vi "Main_2018-02-09.vi"() -> ()   [LabVIEW 2017, in "Client.lvlib"]
uses:
  Client.lvlib
  ClientErrorHandler/ErrorLoopInitData.ctl
  ServerCommunications/TypeDefs/ClientConfiguration.ctl
  ParserSorter/SR Data.ctl
  ParserSorter/AE Group.ctl
  ParserSorter/SR Status.ctl
  ParserSorter/SR Level.ctl
  ParserSorter/SR Type.ctl
  CommunicationsFrameWork/TypeDefs/InternalData.ctl
  ServerCommunications/TypeDefs/SR List.ctl
  ServerCommunications/TypeDefs/SR Data.ctl
  ServerCommunications/TypeDefs/Connection Status.ctl
  UI_API/UIReferences.ctl
  UI_API/SR Fields.ctl
  CommunicationsFrameWork/CommsFrameWork.lvlib
  ServerCommunications/CommsServer.lvlib
  <vilib>/httpClient/LabVIEWHTTPClient.lvlib
  ClientErrorHandler/ClientErrorHandler.lvlib
  ClientLogger/ClientLogger.lvlib
  ParserSorter/ParserSorter.lvlib
  UI_API/UI_API.lvlib
panel:
  out "Prio 4":u32(colorbox)
  out "Prio 3":u32(colorbox)
  out "Prio 2":u32(colorbox)
  out "Prio 1":u32(colorbox)
  in  "Filter Preset":T1(ring)
  out "Time to Refresh":dbl(slide) scale=0.0..10.0
  out "Connection Quality":dbl(knob) scale=0.0..10.0
  out "Connected?":bool
  out "Last Update":timestamp
  in  "Refresh":bool
  in  "AE Level":enum16{"AE / ELP", "AE Intern"}(ring)
  in  "AE Groups":i32[](listbox)
  in  "SRs Tab":enum32{"Unassigned", "Assigned", "Debug"}(tab)
  out "Unassigned Sorted SRs":string[][](table)
  out "Assigned Sorted SRs":string[][](table)
  out "Last Error":errorcluster
  in  "Text":string="Manual Log Entry"
  in  "Type":string="Event"
  in  "Generate Log Entry":bool
  in  "Injected Error":errorcluster
  in  "Generate Error":bool
  # "Priority 1"
  # "Priority 3"
  # "Priority 2"
  # "Priority 4"
  # "Heartbeat Communication"
  # "Manual Loop Control"
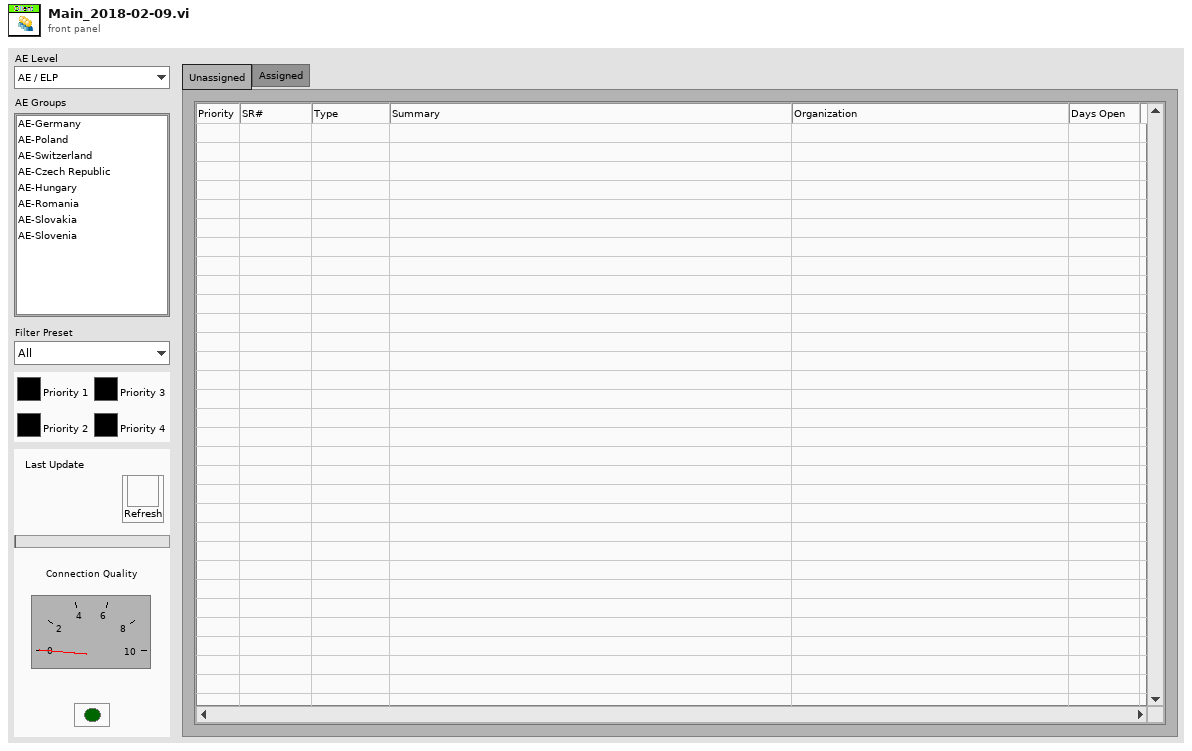
[diagram p1: front panel]
types:
  T1 = enum16{"All", "Eastern Europe", "DACH", "Custom"}
  T2 = typedef "Client.lvlib/CommsFrameWork.lvlib/CommReferences.ctl" = cluster{"ErrorEventReg":refnum<event-registration>, "ErrorEvent":refnum<user-event>, "Queues":cluster{"MHLClient":refnum<queue>, "ErrorHandler":refnum<queue>, "EventHandler":refnum<queue>, "ConnectionHandler":refnum<queue>, "UIHandler":refnum<queue>, "Logger":refnum<queue>}}
  T3 = typedef "LVPoint32TypeDef.ctl" = cluster{"Horizontal":i32, "Vertical":i32}
  T4 = typedef "Client.lvlib/UI_API.lvlib/UIReferences.ctl" = cluster{"Assigned SRs":refnum<vi>, "Unassigned SRs":refnum<vi>, "AE Level":refnum<vi>, "AE Groups":refnum<vi>}
  T5 = typedef "Client.lvlib/ParserSorter.lvlib/SR Data.ctl" = cluster{"SR Number":i64, "AE Group":T6, "SR Owner":string, "Summary":string, "SR Status":T7, "Days Open":dbl, "Prio":T8, "SR Type":T9, "Service Level":string, "Last Updated":timestamp, "First Name":string, "Last Name":string, "Organisation Name":string, "Creation Date":timestamp, "Needs Merging?":bool, "English Flag?":bool}
  T6 = typedef "Client.lvlib/ParserSorter.lvlib/AE Group.ctl" = enum32{"NaN", "AE-Germany", "AE-Poland", "AE-Switzerland", "AE-Czech Republic", "AE-Hungary", "AE-Romania", "AE-Slovakia", "AE-Slovenia"}
  T7 = typedef "Client.lvlib/ParserSorter.lvlib/SR Status.ctl" = enum32{"NaN", "Caller Abandoned", "Created in Error", "Declined to Purchase Support", "Expired", "Forum Resolved AE", "Forum Resolved Customer", "IN WORK", "IN WORK Collab with AES", "IN WORK Collab with PSE", "IN WORK Collab with SE", "IN WORK Escalation", "IN WORK Customer Added Note", "Open", "Potentially Resolved", "POC Resolved", "Resolved", "RMA Waiting on Customer", "RMA Open", "RMA In Progress", "RMA Closed - DOA", "RMA Closed", "RMA Approved for Return", "Project Complete", "Presumed Resolved", "IN WORK Wait on Customer"}
  T8 = typedef "Client.lvlib/ParserSorter.lvlib/SR Level.ctl" = enum16{"Prio 1", "Prio 2", "Prio 3", "Prio 4"}
  T9 = typedef "Client.lvlib/ParserSorter.lvlib/SR Type.ctl" = enum32{"NaN", "ATE Core Configurations (BYOATE)", "Activation", "BioBench", "CAN", "CM C Series", "Calibration", "Consulting Services", "CounterTimer", "DAQExpress", "DASYLab", "DIAdem", "DMM", "DSA HW", "Digital_IO", "FIRST (NIC Only)", "FieldBus", "FieldPoint", "Functional Savety", "GATI", "GPIB", "HMI and Industrial PCs", "HiQ", "HighSpeedDigital_IO", "IMAQ", "IOTech Vibration", "Industrial Communications", "InsightCM", "LV", "LV CD&Sim", "LV Comms", "LV Controls Add-Ons", "LV Embedded", "LV MathScript RT", "LV NXG", "LV NXT", "LVDSC", "LVFPGA", "LVPDA and LV Touch Panel", "LVRT", "LabWindows_CVI", "Lookout", "MATRIXx", "MStudioDotNet", "MStudioVisualBasic", "MStudioVisualC", "Measure (Legacy)", "Motion", "MultifunctionDAQ", "Multimedia Test HW/SW", "Multisim (EWB)", "NI Update Service", "OPC Servers", "Optical (OSI)", "PXI Controllers, Chassis, MXI", "PXI Timing and Sync", "Power Supplies and SMUs", "Powertrain Controls", "RAID", "RF", "RF Software", "RIO", "SC Express", "SCC", "SCXI", "SPEEDY-33 (Hyperception)", "STS", "ScopeDigitizers", "Serial", "Signal Sources", "SignalCondOther", "SignalExpress", "Software Defined Intruments", "Sound and Vibration SW", "Switch Executive", "Switches", "TestStand", "USRP", "Ultiboard (EWB)", "VBench", "VI Logger", "VXI_MXI", "VeriStand", "VisionSW", "VolumeLicenseMgr", "WSN", "Web UI Builder", "myRIO"}
  T10 = typedef "Client.lvlib/CommsServer.lvlib/Connection Status.ctl" = cluster{"Connection Quality":dbl, "Last Update":timestamp}
  T11 = typedef "Client.lvlib/ParserSorter.lvlib/SR Fields.ctl" = enum16{"SR Number", "AE Group", "SR Owner", "Summary", "SR Status", "Days Open", "Prio", "SR Type", "Service Level", "Last Updated", "First Name", "Last Name", "Organisation Name", "Creation Date", "Needs Merging?", "English Flag?"}
  T12 = typedef "Client.lvlib/CommsServer.lvlib/ClientConfiguration.ctl" = cluster{"ColorCodes":u32[]}
  T13 = typedef "Client.lvlib/ClientErrorHandler.lvlib/ErrorLoopInitData.ctl" = cluster{"ErrorsToIgnore":i32[]}
  T14 = typedef "Client.lvlib/CommsFrameWork.lvlib/InternalData.ctl" = cluster{"Connection Data":cluster{"IP":string, "Port":string, "ClientName":string}}
  T15 = typedef "Client.lvlib/CommsServer.lvlib/SR List.ctl" = T16[]
  T16 = typedef "Client.lvlib/CommsServer.lvlib/SR Data.ctl" = cluster{"SR#":dbl, "Group":string, "Owner":string, "Problem Summary":string, "Last Updated":timestamp, "Customer First Name":string, "Customer Last Name":string, "Company":string, "Created On":timestamp, "SR Type":string, "Status":string, "Service Level":string, "Channel":string, "Days Open":dbl}
  T17 = cluster{"IP":string, "Port":string, "ClientName":string}
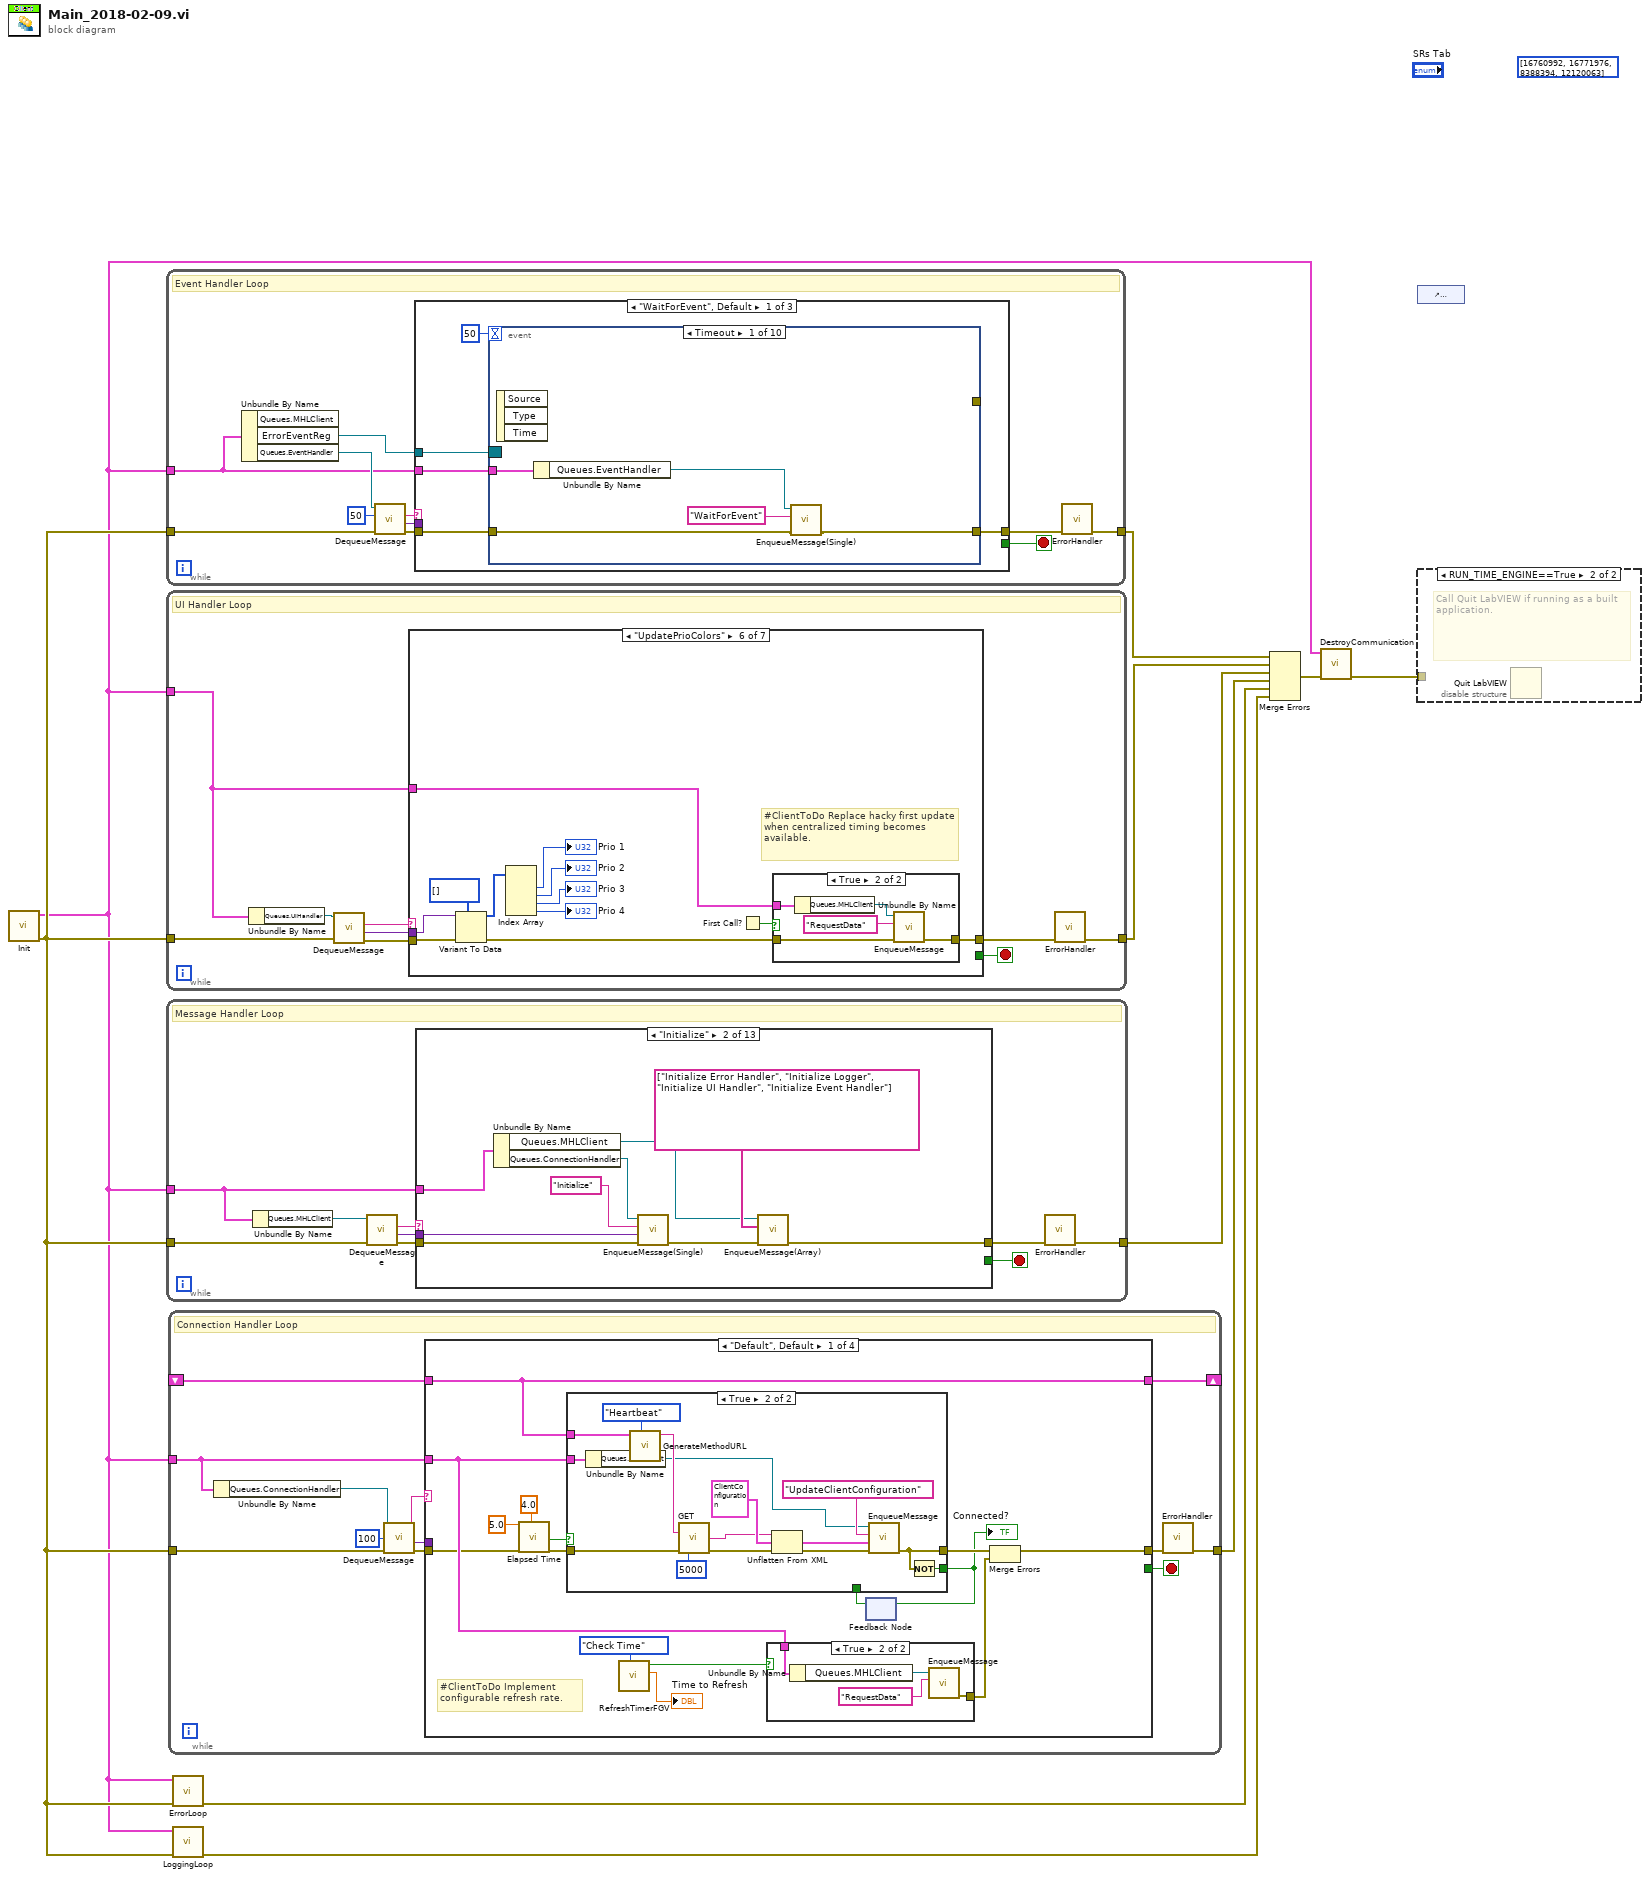
[diagram p0: block diagram]
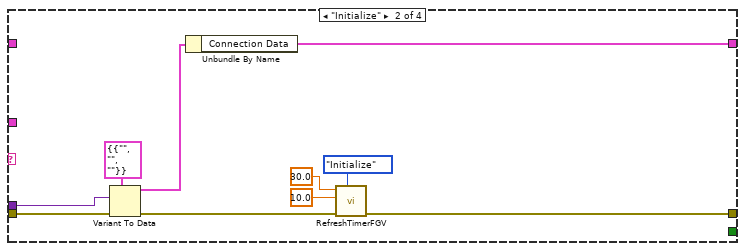
[diagram p4: hidden frame]
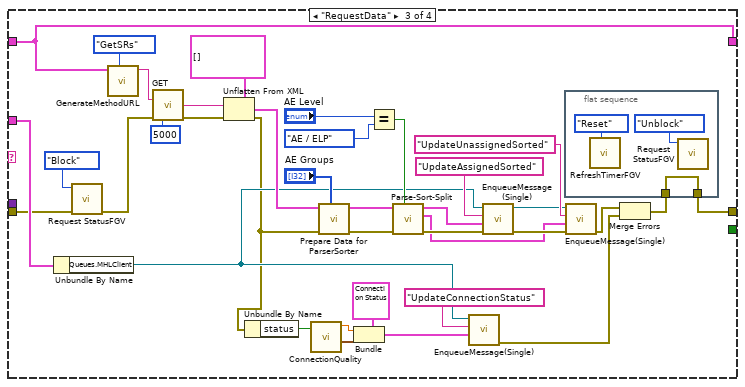
[diagram p5: hidden frame]
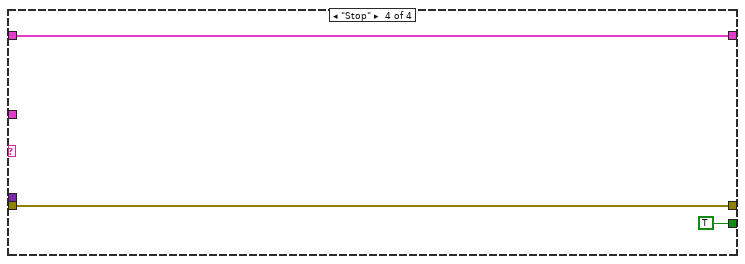
[diagram p6: hidden frame]
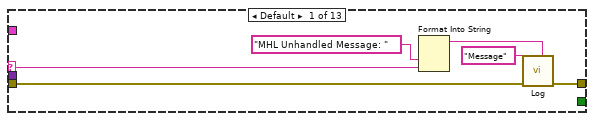
[diagram p7: hidden frame]
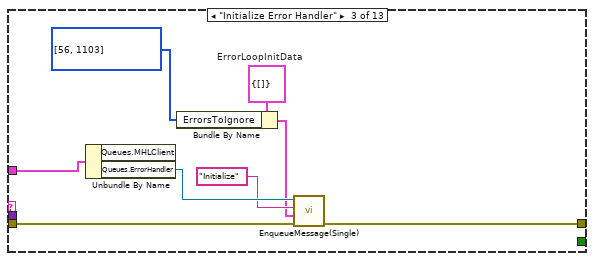
[diagram p8: hidden frame]
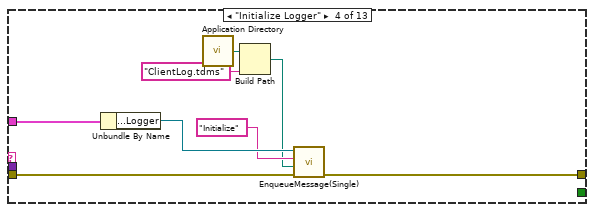
[diagram p9: hidden frame]
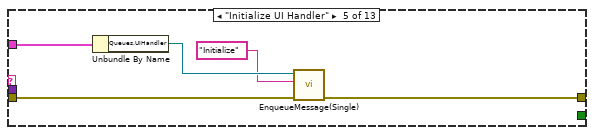
[diagram p10: hidden frame]
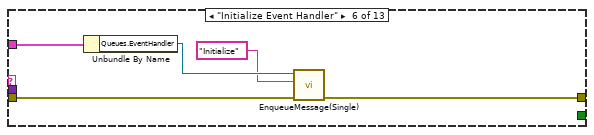
[diagram p11: hidden frame]
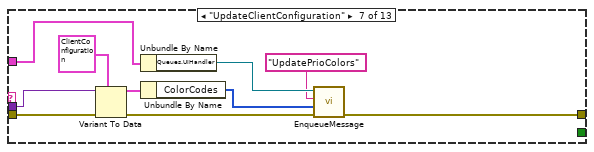
[diagram p12: hidden frame]
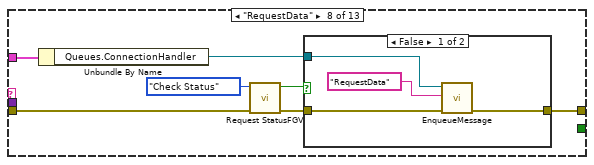
[diagram p13: hidden frame]
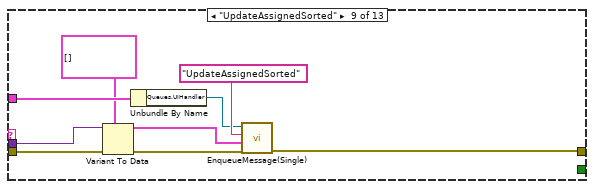
[diagram p15: hidden frame]
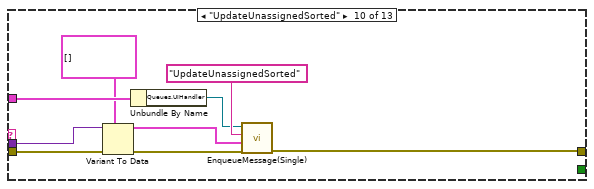
[diagram p16: hidden frame]
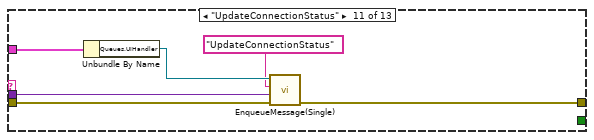
[diagram p17: hidden frame]
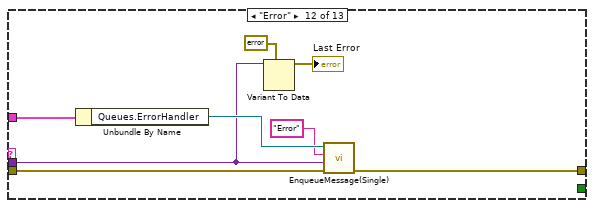
[diagram p18: hidden frame]
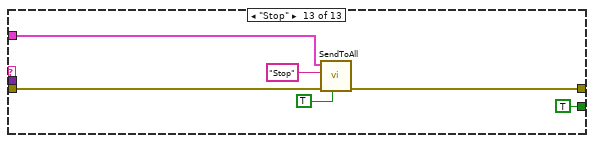
[diagram p19: hidden frame]
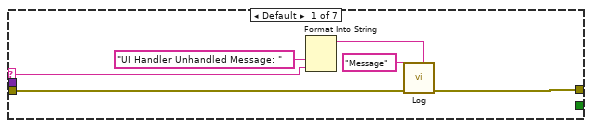
[diagram p20: hidden frame]
diagram:
  (unwired) u32[] [16760992, 16771976, 8388394, 12120063] ("Array")
  n1 = call "Init.vi"() -> ("Error Out"=w4:errorcluster, "Message Queues"=w3:T2)  [unwired: 10 in]
  n2 = while {
    tunnel: w3 -> [w13]
    tunnel: w4 -> [w20]
    tunnel: [w14] -> w9
    stop <- w16 stop-if-true
    # "Event Handler Loop"
    n3 = Unbundle By Name(w13) -> ("ErrorEventReg"=w12:refnum<event-registration>, "Queues.EventHandler"=w21:refnum<queue>)  [unwired: 1 out]
    n4 = call "DequeueMessage.vi"("error in (no error)"=w20, "timeout ms (-1)"=50, "Message Queue"=w21) -> ("error out"=w18:errorcluster, "Message Data"=w17:variant, "Message"=w19:string)  [unwired: 4 in, 2 out]
    n5 = case shown="\"WaitForEvent\", Default" w19 {
      tunnel: w18 -> [w26 w121 w124]
      tunnel: [w23 w120 w124] -> w15
      tunnel: w17 -> [_ _ _]
      tunnel: [_ _ TRUE] -> w16
      tunnel: w13 -> [w25 w119 _]
      tunnel: w12 -> [w22 _ _]
      frame "WaitForEvent", Default {
        n6 = event shown="[0] Timeout" {
          selector: w22 -> [_ _ _ _ _ _ _ _ _ _]
          dyn-events: _ -> [_ _ _ _ _ _ _ _ _ _]
          timeout: 50 -> [_ _ _ _ _ _ _ _ _ _]
          tunnel: w26 -> [w29 w35 w48 w60 w62 w69 w73 w81 w98 w104]
          tunnel: w25 -> [w31 w37 w56 _ _ w68 w75 _ w101 _]
          tunnel: [w30 w33 w49 w60 w61 w65 w72 w80 w99 w103] -> w23
          tunnel: [_ _ _ _ _ _ w70 _ _ _] -> _
          event Timeout {
            n7 = event-data() -> ()  [unwired: 1 in, 3 out]
            n8 = Unbundle By Name(w31) -> ("Queues.EventHandler"=w27:refnum<queue>)
            n9 = call "EnqueueMessage(Single).vi"("error in (no error)"=w29, "Message"="WaitForEvent", "Message Queue"=w27) -> ("error out"=w30:errorcluster)  [unwired: 7 in, 1 out]
          }
          event "Filter Preset": Value Change {
            # "#ClientToDo Replace hardwired values with configuration data."
            n10 = event-data() -> ("NewVal"=w38:T1)  [unwired: 1 in]
            n11 = case shown="\"Eastern Europe\"" w38 {
              tunnel: w35 -> [w39 w41 w43 w45]
              tunnel: [w39 w41 w43 w45] -> w34
              frame "All", Default {
                n12 = property on="AE Groups" class="LstBox (strict)"("Value"=i32[] [0, 1, 2, 3, 4, 5, 6, 7] ("Value (Signaling)")) -> ()  [unwired: 2 in, 2 out]
              }
              frame "Eastern Europe" {
                n13 = property on="AE Groups" class="LstBox (strict)"("Value"=i32[] [1, 3, 4, 5, 6, 7] ("Value (Signaling)")) -> ()  [unwired: 2 in, 2 out]
              }
              frame "DACH" {
                n14 = property on="AE Groups" class="LstBox (strict)"("Value"=i32[] [0, 2] ("Value (Signaling)")) -> ()  [unwired: 2 in, 2 out]
              }
              frame "Custom" {
              }
            }
            n15 = Unbundle By Name(w37) -> ("Queues.MHLClient"=w36:refnum<queue>)
            n16 = call "EnqueueMessage(Single).vi"("error in (no error)"=w34, "Message"="RequestData", "Message Queue"=w36) -> ("error out"=w33:errorcluster)  [unwired: 7 in, 1 out]
          }
          event "AE Level", "AE Groups": Value Change {
            n17 = event-data() -> ("CtlRef"=w54:refnum<vi>)  [unwired: 1 in]
            n18 = call "StopPanelUpdates.vi"("Error In"=w48) -> ("Error Out"=w47:errorcluster)  [unwired: 10 in]
            n19 = property class="Ctl"(reference=w54) -> ("Label.Text"=w53:string)  [unwired: 1 in, 2 out]
            n20 = Unbundle By Name(w56) -> ("Queues.MHLClient"=w57:refnum<queue>)
            n21 = case shown="\"AE Groups\"" w53 {
              frame "False", Default {
              }
              frame "AE Groups" {
                n22 = local write "Filter Preset"(T1."Custom" ("Filter Preset")) -> ()
              }
            }
            n23 = call "EnqueueMessage(Single).vi"("error in (no error)"=w47, "Message"="RequestData", "Message Queue"=w57) -> ("error out"=w46:errorcluster)  [unwired: 7 in, 1 out]
            n24 = control-ref of="Unassigned Sorted SRs"() -> (w52:refnum<vi>)
            n25 = control-ref of="Assigned Sorted SRs"() -> (w51:refnum<vi>)
            n26 = Build Array(w52, w51) -> (w50:refnum<vi>[])
            n27 = call "ResetTablesToTopPosition.vi"("Error In"=w46, "Table Refnum Array"=w50) -> ("Error Out"=w49:errorcluster)  [unwired: 9 in]
          }
          event "Generate Error": Value Change {
            n28 = event-data() -> ()  [unwired: 1 in, 6 out]
            n29 = call "ErrorHandler.vi"("error in (no error)"="Injected Error") -> ()  [unwired: 10 in, 1 out]
          }
          event "Generate Log Entry": Value Change {
            n30 = event-data() -> ()  [unwired: 1 in, 6 out]
            n31 = call "Log.vi"("LogMessage"="Text", "Type"="Type", "Error In"=w62) -> ("Error Out"=w61:errorcluster)  [unwired: 8 in]
          }
          event "Refresh": Value Change {
            n32 = event-data() -> ()  [unwired: 1 in, 1 out]
            n33 = Unbundle By Name(w68) -> ("Queues.MHLClient"=w67:refnum<queue>)
            n34 = call-poly "EnqueueMessage.vi"("error in (no error)"=w69, "Message"="RequestData", "Message Queue"=w67) -> ("error out"=w65:errorcluster)  [unwired: 7 in, 1 out]
          }
          event User Event {
            n35 = event-data() -> ("status"=w78:bool, "code"=w77:i32, "source"=w76:string)  [unwired: 1 in]
            n36 = Unbundle By Name(w75) -> ("Queues.MHLClient"=w74:refnum<queue>)
            n37 = Bundle(cluster=errorcluster {"status"=FALSE, "code"=0, "source"=""} ("error constant"), "status"=w78, "code"=w77, "source"=w76) -> (w70:errorcluster)
            n38 = call "EnqueueMessage(Single).vi"("error in (no error)"=w73, "Message"="Stop", "Message Queue"=w74) -> ("error out"=w72:errorcluster)  [unwired: 7 in, 1 out]
          }
          event "Unassigned Sorted SRs": Shortcut Menu Selection (User) {
            # "#ClientToDo Adapt SR# finding to configurable columns"
            n39 = event-data() -> ("ItemTag"=w82:string, "CtlRef"=w84:refnum<vi>, "Coords"=w83:T3)  [unwired: 1 in]
            n40 = case shown="\"Copy SR#\", Default" w82 {
              tunnel: w84 -> [w90 w95]
              tunnel: w83 -> [w89 w93]
              tunnel: [w85 w92] -> w80
              tunnel: w81 -> [w86 w91]
              frame "Open Screenpop" {
                # "#ClientToDo URL from config data."
                n41 = call "Open Screenpop.vi"("Screenpop URL Prefix"="http://force.natinst.com:8000/pls/ebiz/niae_screenpop.main?p_incident_number=", "SR# Cloumn Header"="SR#" ("SR Cloumn Header"), "Error In"=w86, "Coordinates"=w89, "Table Reference"=w90) -> ("Error Out"=w85:errorcluster)  [unwired: 6 in]
              }
              frame "Copy SR#", Default {
                n42 = call "Copy SR Num to Clipboard.vi"("SR Cloumn Header"="SR#", "Error In"=w91, "Coordinates"=w93, "Table Reference"=w95) -> ("Error Out"=w92:errorcluster)  [unwired: 7 in]
              }
            }
          }
          event Panel Close? {
            n43 = event-data() -> ()  [unwired: 1 in, 1 out]
            n44 = Unbundle By Name(w101) -> ("Queues.MHLClient"=w100:refnum<queue>)
            n45 = call "EnqueueMessage(Single).vi"("Priority Message? (F)"=TRUE, "error in (no error)"=w98, "Message"="Stop", "Message Queue"=w100) -> ("error out"=w99:errorcluster)  [unwired: 6 in, 1 out]
            n46 = event-data("Discard?"=TRUE) -> ()  [unwired: 1 in, 1 out]
          }
          event "Assigned Sorted SRs": Shortcut Menu Selection (User) {
            # "#ClientToDo Adapt SR# finding to configurable columns"
            n47 = event-data() -> ("ItemTag"=w107:string, "CtlRef"=w106:refnum<vi>, "Coords"=w105:T3)  [unwired: 1 in]
            n48 = case shown="\"Open Screenpop\"" w107 {
              tunnel: w106 -> [w113 w118]
              tunnel: w105 -> [w112 w116]
              tunnel: w104 -> [w109 w115]
              tunnel: [w108 w114] -> w103
              frame "Open Screenpop" {
                # "#ClientToDo URL from config data."
                n49 = call "Open Screenpop.vi"("Screenpop URL Prefix"="http://force.natinst.com:8000/pls/ebiz/niae_screenpop.main?p_incident_number=", "SR# Cloumn Header"="SR#" ("SR Cloumn Header"), "Error In"=w109, "Coordinates"=w112, "Table Reference"=w113) -> ("Error Out"=w108:errorcluster)  [unwired: 6 in]
              }
              frame "Copy SR#", Default {
                n50 = call "Copy SR Num to Clipboard.vi"("SR Cloumn Header"="SR#", "Error In"=w115, "Coordinates"=w116, "Table Reference"=w118) -> ("Error Out"=w114:errorcluster)  [unwired: 7 in]
              }
            }
          }
        }
      }
      frame "Initialize" {
        n51 = Unbundle By Name(w119) -> ("Queues.EventHandler"=w123:refnum<queue>)
        n52 = call "EnqueueMessage(Single).vi"("error in (no error)"=w121, "Message"="WaitForEvent", "Message Queue"=w123) -> ("error out"=w120:errorcluster)  [unwired: 7 in, 1 out]
      }
      frame "Stop" {
      }
    }
    n53 = call "ErrorHandler.vi"("error in (no error)"=w15) -> ("error out"=w14:errorcluster)  [unwired: 10 in]
  }
  n54 = while {
    tunnel: w3 -> [w128]
    tunnel: w4 -> [w133]
    tunnel: [w126] -> w8
    stop <- w129 stop-if-true
    # "UI Handler Loop"
    n55 = Unbundle By Name(w128) -> ("Queues.UIHandler"=w134:refnum<queue>)
    n56 = call "DequeueMessage.vi"("error in (no error)"=w133, "Message Queue"=w134) -> ("error out"=w132:errorcluster, "Message Data"=w130:variant, "Message"=w131:string)  [unwired: 5 in, 2 out]
    n57 = case shown="\"UpdatePrioColors\"" w131 {
      selector: w131 -> [w137 _ _ _ _ _ _]
      tunnel: w132 -> [w136 w145 w169 w185 w195 w206 w215]
      tunnel: [w135 w141 w153 w172 w194 w196 w214] -> w127
      tunnel: w130 -> [_ _ w170 w186 w193 w205 _]
      tunnel: [_ _ _ _ _ _ TRUE] -> w129
      tunnel: w128 -> [_ _ _ _ _ w198 _]
      frame Default {
        n58 = Format Into String("UI Handler Unhandled Message: " ("Type"), w137) -> (resulting string=w140:string)  [unwired: 3 in, 1 out]
        n59 = call "Log.vi"("LogMessage"=w140, "Type"="Message", "Error In"=w136) -> ("Error Out"=w135:errorcluster)  [unwired: 8 in]
      }
      frame "Initialize" {
        n60 = call "StopPanelUpdates.vi"("Error In"=w145) -> ("Error Out"=w144:errorcluster)  [unwired: 10 in]
        n61 = control-ref of="AE Groups"() -> (w148:refnum<vi>)
        n62 = control-ref of="AE Level"() -> (w150:refnum<vi>)
        n63 = control-ref of="Unassigned Sorted SRs"() -> (w151:refnum<vi>)
        n64 = control-ref of="Assigned Sorted SRs"() -> (w152:refnum<vi>)
        n65 = call "InitAE-Groups.vi"("Error In"=w144, "LstBox Refnum"=w148) -> ("Error Out"=w147:errorcluster)  [unwired: 9 in]
        n66 = Bundle(cluster=T4 {"Assigned SRs"=refnum, "Unassigned SRs"=refnum, "AE Level"=refnum, "AE Groups"=refnum} ("UI References"), "Assigned SRs"=w152, "Unassigned SRs"=w151, "AE Level"=w150, "AE Groups"=w148) -> (w146:T4)
        n67 = call "RestoreUISettings.vi"("Error In"=w147, "UI References"=w146) -> ("Error Out"=w143:errorcluster)  [unwired: 9 in]
        n68 = call "StartPanelUpdates.vi"("Ignore Error In"=TRUE, "Error In"=w143) -> ("Error Out"=w141:errorcluster)  [unwired: 9 in]
      }
      frame "UpdateAssignedSorted" {
        w167 = T11[] [enum."SR Owner", enum."SR Number", enum."Summary", enum."Organisation Name"] items=["SR Number", "AE Group", "SR Owner", "Summary", "SR Status", "Days Open", "Prio", "SR Type", "Service Level", "Last Updated", "First Name", "Last Name", "Organisation Name", "Creation Date", "Needs Merging?", "English Flag?"] ("Fields to include")
        # "#ClientToDo Implement configurable columns."
        n69 = Variant To Data(error in=w169, type=T5[] [] ("SR List In"), Variant=w170) -> (data=w164:T5[], error out=w157:errorcluster)
        n70 = call "StopPanelUpdates.vi"("Error In"=w157) -> ("Error Out"=w156:errorcluster)  [unwired: 10 in]
        n71 = call "SRListToTable.vi"("Fields to include"=w167, "Error In"=w156, "SR List In"=w164) -> ("Error Out"=w165:errorcluster, "2D String Array for Table"=→"Assigned Sorted SRs":string[][])  [unwired: 7 in]
        n72 = local read "Prio 1"() -> (w162:u32)
        n73 = local read "Prio 2"() -> (w161:u32)
        n74 = local read "Prio 3"() -> (w160:u32)
        n75 = local read "Prio 4"() -> (w159:u32)
        n76 = control-ref of="Assigned Sorted SRs"() -> (w163:refnum<vi>)
        n77 = Build Array(w162, w161, w160, w159) -> (w158:u32[])
        n78 = call "PriorityColoring.vi"("Color Array"=w158, "Error In"=w165, "Tbl Refnum"=w163, "SR List In"=w164) -> ("Error Out"=w155:errorcluster)  [unwired: 7 in]
        n79 = call "StartPanelUpdates.vi"("Ignore Error In"=TRUE, "Error In"=w155) -> ("Error Out"=w153:errorcluster)  [unwired: 9 in]
      }
      frame "UpdateUnassignedSorted" {
        w187 = T11[] [enum."Prio", enum."SR Number", enum."SR Type", enum."Summary", enum."Organisation Name", enum."Days Open", enum."First Name", enum."Last Name"] items=["SR Number", "AE Group", "SR Owner", "Summary", "SR Status", "Days Open", "Prio", "SR Type", "Service Level", "Last Updated", "First Name", "Last Name", "Organisation Name", "Creation Date", "Needs Merging?", "English Flag?"] ("Fields to include")
        # "#ClientToDo Implement configurable columns."
        n80 = Variant To Data(error in=w185, type=T5[] [] ("SR List In"), Variant=w186) -> (data=w182:T5[], error out=w175:errorcluster)
        n81 = call "StopPanelUpdates.vi"("Error In"=w175) -> ("Error Out"=w174:errorcluster)  [unwired: 10 in]
        n82 = call "SRListToTable.vi"("Fields to include"=w187, "Error In"=w174, "SR List In"=w182) -> ("Error Out"=w183:errorcluster, "2D String Array for Table"=→"Unassigned Sorted SRs":string[][])  [unwired: 7 in]
        n83 = local read "Prio 1"() -> (w180:u32)
        n84 = local read "Prio 2"() -> (w179:u32)
        n85 = local read "Prio 3"() -> (w178:u32)
        n86 = local read "Prio 4"() -> (w177:u32)
        n87 = control-ref of="Unassigned Sorted SRs"() -> (w181:refnum<vi>)
        n88 = Build Array(w180, w179, w178, w177) -> (w176:u32[])
        n89 = call "PriorityColoring.vi"("Color Array"=w176, "Error In"=w183, "Tbl Refnum"=w181, "SR List In"=w182) -> ("Error Out"=w173:errorcluster)  [unwired: 7 in]
        n90 = call "StartPanelUpdates.vi"("Ignore Error In"=TRUE, "Error In"=w173) -> ("Error Out"=w172:errorcluster)  [unwired: 9 in]
      }
      frame "UpdateConnectionStatus" {
        n91 = Variant To Data(error in=w195, type=T10 {"Connection Quality"=0.0, "Last Update"=timestamp(0 s since 1904-01-01)} ("Connection Status"), Variant=w193) -> (data=w191:T10, error out=w194:errorcluster)
        n92 = Unbundle(w191) -> ("Connection Quality"=→"Connection Quality":dbl, "Last Update"=→"Last Update":timestamp)
      }
      frame "UpdatePrioColors" {
        # "#ClientToDo Replace hacky first update when centralized timing becomes available."
        n93 = Variant To Data(error in=w206, type=u32[] [] ("ColorCodes"), Variant=w205) -> (data=w204:u32[], error out=w197:errorcluster)
        n94 = Index Array(array=w204) -> (element #1=→"Prio 1":u32, element #2=→"Prio 2":u32, element #3=→"Prio 3":u32, element #4=→"Prio 4":u32)  [unwired: 4 in]
        n95 = First Call?() -> (First Call?: T/F=w199:bool)
        n96 = case shown="True" w199 {
          tunnel: w198 -> [_ w212]
          tunnel: w197 -> [w208 w210]
          tunnel: [w208 w209] -> w196
          frame False {
          }
          frame True {
            n97 = Unbundle By Name(w212) -> ("Queues.MHLClient"=w211:refnum<queue>)
            n98 = call-poly "EnqueueMessage.vi"("error in (no error)"=w210, "Message"="RequestData", "Message Queue"=w211) -> ("error out"=w209:errorcluster)  [unwired: 7 in, 1 out]
          }
        }
      }
      frame "Stop" {
        n99 = control-ref of="AE Groups"() -> (w218:refnum<vi>)
        n100 = control-ref of="AE Level"() -> (w219:refnum<vi>)
        n101 = control-ref of="Unassigned Sorted SRs"() -> (w220:refnum<vi>)
        n102 = control-ref of="Assigned Sorted SRs"() -> (w221:refnum<vi>)
        n103 = Bundle(cluster=T4 {"Assigned SRs"=refnum, "Unassigned SRs"=refnum, "AE Level"=refnum, "AE Groups"=refnum} ("UI References"), "Assigned SRs"=w221, "Unassigned SRs"=w220, "AE Level"=w219, "AE Groups"=w218) -> (w216:T4)
        n104 = call "SaveUISettings.vi"("Error In"=w215, "UI References"=w216) -> ("Error Out"=w214:errorcluster)  [unwired: 9 in]
      }
    }
    n105 = call "ErrorHandler.vi"("error in (no error)"=w127) -> ("error out"=w126:errorcluster)  [unwired: 10 in]
  }
  n106 = while {
    tunnel: w3 -> [w225]
    tunnel: w4 -> [w231]
    tunnel: [w223] -> w7
    stop <- w226 stop-if-true
    # "Message Handler Loop"
    n107 = Unbundle By Name(w225) -> ("Queues.MHLClient"=w230:refnum<queue>)
    n108 = call "DequeueMessage.vi"("error in (no error)"=w231, "Message Queue"=w230) -> ("error out"=w227:errorcluster, "Message Data"=w228:variant, "Message"=w229:string)  [unwired: 5 in, 2 out]
    n109 = case shown="\"Initialize\"" w229 {
      selector: w229 -> [w236 _ _ _ _ _ _ _ _ _ _ _ _]
      tunnel: w228 -> [_ w246 _ _ _ _ w281 _ w301 w310 w316 w321 _]
      tunnel: w227 -> [w233 w243 w253 w261 w266 w271 w282 w285 w300 w309 w318 w323 w330]
      tunnel: [w232 w239 w250 w258 w263 w268 w277 w289 w295 w304 w317 w322 w329] -> w224
      tunnel: [_ _ _ _ _ _ _ _ _ _ _ _ TRUE] -> w226
      tunnel: w225 -> [_ w245 w254 w262 w267 w272 w275 w288 w303 w312 w315 w326 w328]
      frame Default {
        n110 = Format Into String("MHL Unhandled Message: " ("Type"), w236) -> (resulting string=w234:string)  [unwired: 3 in, 1 out]
        n111 = call "Log.vi"("LogMessage"=w234, "Type"="Message", "Error In"=w233) -> ("Error Out"=w232:errorcluster)  [unwired: 8 in]
      }
      frame "Initialize" {
        n112 = Unbundle By Name(w245) -> ("Queues.MHLClient"=w238:refnum<queue>, "Queues.ConnectionHandler"=w244:refnum<queue>)
        n113 = call "EnqueueMessage(Single).vi"("error in (no error)"=w243, "Message Data"=w246, "Message"="Initialize", "Message Queue"=w244) -> ("error out"=w241:errorcluster)  [unwired: 6 in, 1 out]
        n114 = call "EnqueueMessage(Array).vi"("error in (no error)"=w241, "Message Array"=string[] ["Initialize Error Handler", "Initialize Logger", "Initialize UI Handler", "Initialize Event Handler"], "Message Queue"=w238) -> ("error out"=w239:errorcluster)  [unwired: 7 in, 1 out]
      }
      frame "Initialize Error Handler" {
        w249 = T13 {"ErrorsToIgnore"=[]}  # ErrorLoopInitData
        n115 = Unbundle By Name(w254) -> ("Queues.ErrorHandler"=w252:refnum<queue>)  [unwired: 1 out]
        n116 = Bundle By Name(cluster=w249, "ErrorsToIgnore"=i32[] [56, 1103]) -> (w248:T13)
        n117 = call "EnqueueMessage(Single).vi"("error in (no error)"=w253, "Message Data"=w248, "Message"="Initialize", "Message Queue"=w252) -> ("error out"=w250:errorcluster)  [unwired: 6 in, 1 out]
      }
      frame "Initialize Logger" {
        n118 = Unbundle By Name(w262) -> ("Queues.Logger"=w260:refnum<queue>)
        n119 = call <vilib>:"Application Directory.vi"() -> ("Application Directory"=w257:path)
        n120 = Build Path(base path=w257, name or relative path="ClientLog.tdms") -> (appended path=w255:path)
        n121 = call "EnqueueMessage(Single).vi"("error in (no error)"=w261, "Message Data"=w255, "Message"="Initialize", "Message Queue"=w260) -> ("error out"=w258:errorcluster)  [unwired: 6 in, 1 out]
      }
      frame "Initialize UI Handler" {
        n122 = Unbundle By Name(w267) -> ("Queues.UIHandler"=w265:refnum<queue>)
        n123 = call "EnqueueMessage(Single).vi"("error in (no error)"=w266, "Message"="Initialize", "Message Queue"=w265) -> ("error out"=w263:errorcluster)  [unwired: 7 in, 1 out]
      }
      frame "Initialize Event Handler" {
        n124 = Unbundle By Name(w272) -> ("Queues.EventHandler"=w270:refnum<queue>)
        n125 = call "EnqueueMessage(Single).vi"("error in (no error)"=w271, "Message"="Initialize", "Message Queue"=w270) -> ("error out"=w268:errorcluster)  [unwired: 7 in, 1 out]
      }
      frame "UpdateClientConfiguration" {
        n126 = Variant To Data(error in=w282, type=T12 {"ColorCodes"=[16711680, 6618880, 16774745, 9567230]} ("ClientConfig"), Variant=w281) -> (data=w279:T12, error out=w278:errorcluster)
        n127 = Unbundle By Name(w275) -> ("Queues.UIHandler"=w274:refnum<queue>)
        n128 = Unbundle By Name(w279) -> ("ColorCodes"=w276:u32[])
        n129 = call-poly "EnqueueMessage.vi"("error in (no error)"=w278, "Message Data"=w276, "Message"="UpdatePrioColors", "Message Queue"=w274) -> ("error out"=w277:errorcluster)  [unwired: 6 in, 1 out]
      }
      frame "RequestData" {
        n130 = Unbundle By Name(w288) -> ("Queues.ConnectionHandler"=w287:refnum<queue>)
        n131 = call "Request StatusFGV.vi"("Error In"=w285, "Command"=enum16{"Block", "Unblock", "Check Status"}."Check Status") -> ("Error Out"=w284:errorcluster, "Blocked?"=w283:bool)  [unwired: 8 in]
        n132 = case shown="False" w283 {
          tunnel: [w293 w294] -> w289
          tunnel: w287 -> [w292 _]
          tunnel: w284 -> [w290 w294]
          frame False {
            n133 = call-poly "EnqueueMessage.vi"("error in (no error)"=w290, "Message"="RequestData", "Message Queue"=w292) -> ("error out"=w293:errorcluster)  [unwired: 7 in, 1 out]
          }
          frame True {
          }
        }
      }
      frame "UpdateAssignedSorted" {
        n134 = Variant To Data(error in=w300, type=T5[] [] ("SR List In"), Variant=w301) -> (data=w297:T5[], error out=w296:errorcluster)
        n135 = Unbundle By Name(w303) -> ("Queues.UIHandler"=w299:refnum<queue>)
        n136 = call "EnqueueMessage(Single).vi"("error in (no error)"=w296, "Message Data"=w297, "Message"="UpdateAssignedSorted", "Message Queue"=w299) -> ("error out"=w295:errorcluster)  [unwired: 6 in, 1 out]
      }
      frame "UpdateUnassignedSorted" {
        n137 = Variant To Data(error in=w309, type=T5[] [] ("SR List In"), Variant=w310) -> (data=w306:T5[], error out=w305:errorcluster)
        n138 = Unbundle By Name(w312) -> ("Queues.UIHandler"=w308:refnum<queue>)
        n139 = call "EnqueueMessage(Single).vi"("error in (no error)"=w305, "Message Data"=w306, "Message"="UpdateUnassignedSorted", "Message Queue"=w308) -> ("error out"=w304:errorcluster)  [unwired: 6 in, 1 out]
      }
      frame "UpdateConnectionStatus" {
        n140 = Unbundle By Name(w315) -> ("Queues.UIHandler"=w314:refnum<queue>)
        n141 = call "EnqueueMessage(Single).vi"("error in (no error)"=w318, "Message Data"=w316, "Message"="UpdateConnectionStatus", "Message Queue"=w314) -> ("error out"=w317:errorcluster)  [unwired: 6 in, 1 out]
      }
      frame "Error" {
        n142 = Unbundle By Name(w326) -> ("Queues.ErrorHandler"=w325:refnum<queue>)
        n143 = Variant To Data(type=errorcluster {"status"=FALSE, "code"=0, "source"=""} ("error constant"), Variant=w321) -> (data=→"Last Error":errorcluster)  [unwired: 1 in, 1 out]
        n144 = call "EnqueueMessage(Single).vi"("error in (no error)"=w323, "Message Data"=w321, "Message"="Error", "Message Queue"=w325) -> ("error out"=w322:errorcluster)  [unwired: 6 in, 1 out]
      }
      frame "Stop" {
        n145 = call "SendToAll.vi"("Priority Message? (F)"=TRUE, "error in (no error)"=w330, "Message"="Stop", "Message Queues"=w328) -> ("error out"=w329:errorcluster)  [unwired: 7 in]
      }
    }
    n146 = call "ErrorHandler.vi"("error in (no error)"=w224) -> ("error out"=w223:errorcluster)  [unwired: 10 in]
  }
  n147 = while {
    tunnel: w3 -> [w338]
    shift-right: [w336] -> _
    shift-left: _ -> [w335]
    tunnel: w4 -> [w344]
    tunnel: [w333] -> w6
    stop <- w339 stop-if-true
    # "Connection Handler Loop"
    n148 = Unbundle By Name(w338) -> ("Queues.ConnectionHandler"=w343:refnum<queue>)
    n149 = call "DequeueMessage.vi"("error in (no error)"=w344, "timeout ms (-1)"=100, "Message Queue"=w343) -> ("error out"=w340:errorcluster, "Message Data"=w341:variant, "Message"=w342:string)  [unwired: 4 in, 2 out]
    n150 = case shown="\"Default\", Default" w342 {
      tunnel: w341 -> [_ w389 _ _]
      tunnel: w340 -> [w350 w390 w399 w432]
      tunnel: [w357 w384 w391 w432] -> w334
      tunnel: [_ _ _ TRUE] -> w339
      tunnel: w338 -> [w353 _ w422 _]
      tunnel: [w359 w386 w427 w431] -> w336
      tunnel: w335 -> [w359 _ w427 w431]
      frame "Default", Default {
        # "#ClientToDo Implement configurable refresh rate."
        n151 = call "Elapsed Time"("Time Target (s)"=5.0, "error in (no error)"=w350, "Set Start Time (s)"=4.0) -> ("Time has Elapsed"=w348:bool, "error out"=w349:errorcluster)  [unwired: 9 in, 6 out]
        n152 = call "RefreshTimerFGV.vi"("Command"=enum16{"Initialize", "Check Time", "Reset"}."Check Time") -> ("Time to Next Refresh"=→"Time to Refresh":dbl, "Refresh Now?"=w347:bool)  [unwired: 8 in, 1 out]
        n153 = case shown="True" w347 {
          tunnel: w353 -> [_ w380]
          tunnel: [_ w377] -> w358
          frame False {
          }
          frame True {
            n154 = Unbundle By Name(w380) -> ("Queues.MHLClient"=w379:refnum<queue>)
            n155 = call-poly "EnqueueMessage.vi"("Message"="RequestData", "Message Queue"=w379) -> ("error out"=w377:errorcluster)  [unwired: 8 in, 1 out]
          }
        }
        n156 = feedback #1() -> (w354:bool)  [unwired: 1 in]
        n157 = case shown="True" w348 {
          tunnel: w359 -> [_ w376]
          tunnel: w349 -> [w361 w374]
          tunnel: [w360 w372] -> w355
          tunnel: [w361 w371] -> w356
          tunnel: w354 -> [w360 _]
          tunnel: w353 -> [_ w369]
          frame False {
          }
          frame True {
            n158 = Unbundle By Name(w369) -> ("Queues.MHLClient"=w363:refnum<queue>)
            n159 = call "GenerateMethodURL.vi"("Method"=enum16{"Heartbeat", "GetSRs"}."Heartbeat", "TestClientData"=w376) -> ("String"=w373:string)  [unwired: 9 in]
            n160 = call <vilib>:"GET.vi"("url"=w373, "error in (no error)"=w374, "timeout (10000)"=5000) -> ("body"=w365:string, "error out"=w368:errorcluster)  [unwired: 9 in, 2 out]
            n161 = Unflatten From XML(xml string=w365, type=T12 {"ColorCodes"=[16711680, 6618880, 16774745, 9567230]} ("ClientConfig"), error in (no error)=w368) -> (value=w364:T12, error out=w367:errorcluster)
            n162 = call-poly "EnqueueMessage.vi"("error in (no error)"=w367, "Message Data"=w364, "Message"="UpdateClientConfiguration", "Message Queue"=w363) -> ("error out"=w371:errorcluster)  [unwired: 6 in, 1 out]
            n163 = Not(x=w371) -> (.not. x?=w372:bool)
          }
        }
        "Connected?" <- w355
        n164 = feedback-in #1(w355) -> ()
        n165 = Merge Errors(w356, w358) -> (w357:errorcluster)
      }
      frame "Initialize" {
        n166 = Variant To Data(error in=w390, type=T14 {"Connection Data"={"IP"="", "Port"="", "ClientName"=""}} ("InternalData"), Variant=w389) -> (data=w387:T14, error out=w385:errorcluster)
        n167 = Unbundle By Name(w387) -> ("Connection Data"=w386:T17)
        n168 = call "RefreshTimerFGV.vi"("Command"=enum16{"Initialize", "Check Time", "Reset"}."Initialize", "Error In"=w385, "Ticker Multiplier"=10.0, "Refresh Period [s]"=30.0) -> ("Error Out"=w384:errorcluster)  [unwired: 5 in, 2 out]
      }
      frame "RequestData" {
        n169 = Unbundle By Name(w422) -> ("Queues.MHLClient"=w401:refnum<queue>)
        n170 = call "Request StatusFGV.vi"("Error In"=w399, "Command"=enum16{"Block", "Unblock", "Check Status"}."Block") -> ("Error Out"=w398:errorcluster)  [unwired: 8 in, 1 out]
        n171 = call "GenerateMethodURL.vi"("Method"=enum16{"Heartbeat", "GetSRs"}."GetSRs", "TestClientData"=w427) -> ("String"=w425:string)  [unwired: 9 in]
        n172 = call <vilib>:"GET.vi"("url"=w425, "error in (no error)"=w398, "timeout (10000)"=5000) -> ("body"=w424:string, "error out"=w394:errorcluster)  [unwired: 9 in, 2 out]
        n173 = Unflatten From XML(xml string=w424, type=T15 [] ("SRList"), error in (no error)=w394) -> (value=w421:T15, error out=w393:errorcluster)
        n174 = Unbundle By Name(w393) -> ("status"=w406:bool)
        n175 = call "ConnectionQuality.vi"("Error?"=w406) -> ("Last Update"=w403:timestamp, "Connection Quality"=w404:dbl)  [unwired: 9 in]
        n176 = call "Prepare Data for ParserSorter.vi"("AE Groups to Include"="AE Groups", "Error In"=w393, "SRList"=w421) -> ("Error Out"=w418:errorcluster, "Prepared SR List"=w419:T5[])  [unwired: 7 in]
        n177 = Bundle(cluster=T10 {"Connection Quality"=0.0, "Last Update"=timestamp(0 s since 1904-01-01)} ("Connection Status"), "Connection Quality"=w404, "Last Update"=w403) -> (w402:T10)
        n178 = Equal?(x="AE Level", y=enum16{"AE / ELP", "AE Intern"}."AE / ELP") -> (x = y?=w416:bool)
        n179 = call "Parse-Sort-Split.vi"("Include High Priority?"=w416, "Error In"=w418, "SR List In"=w419) -> ("Error Out"=w413:errorcluster, "Unassigned SR List"=w410:T5[], "Assigned SR List"=w414:T5[])  [unwired: 6 in]
        n180 = call "EnqueueMessage(Single).vi"("Message Data"=w402, "Message"="UpdateConnectionStatus", "Message Queue"=w401) -> ("error out"=w395:errorcluster)  [unwired: 7 in, 1 out]
        n181 = call "EnqueueMessage(Single).vi"("error in (no error)"=w413, "Message Data"=w414, "Message"="UpdateAssignedSorted", "Message Queue"=w401) -> ("error out"=w412:errorcluster, "dup Message Queue"=w408:refnum<queue>)  [unwired: 6 in]
        n182 = flat-sequence {
          tunnel: w392 -> [w429]
          tunnel: [w429] -> w391
          frame #0 {
            n183 = call "RefreshTimerFGV.vi"("Command"=enum16{"Initialize", "Check Time", "Reset"}."Reset") -> ()  [unwired: 8 in, 3 out]
            n184 = call "Request StatusFGV.vi"("Command"=enum16{"Block", "Unblock", "Check Status"}."Unblock") -> ()  [unwired: 9 in, 2 out]
          }
        }
        n185 = call "EnqueueMessage(Single).vi"("error in (no error)"=w412, "Message Data"=w410, "Message"="UpdateUnassignedSorted", "Message Queue"=w408) -> ("error out"=w411:errorcluster)  [unwired: 6 in, 1 out]
        n186 = Merge Errors(w411, w395) -> (w392:errorcluster)
      }
      frame "Stop" {
      }
    }
    n187 = call "ErrorHandler.vi"("error in (no error)"=w334) -> ("error out"=w333:errorcluster)  [unwired: 10 in]
  }
  n188 = call "ErrorLoop.vi"("Error In"=w4, "Message Queues"=w3) -> ("Error Out"=w5:errorcluster)  [unwired: 9 in]
  n189 = call "LoggingLoop.vi"("Error In"=w4, "Communication References"=w3) -> ("Error Out"=w2:errorcluster)  [unwired: 9 in]
  n190 = Merge Errors(w9, w8, w7, w6, w5, w2) -> (w10:errorcluster)
  n191 = call "DestroyCommunication.vi"("error in (no error)"=w10, "Message Queues"=w3) -> ("error out"=w1:errorcluster)  [unwired: 9 in]
  n192 = control-ref of="Unassigned Sorted SRs"() -> ()  [unwired: 1 out]
  n193 = disable-structure shown="RUN_TIME_ENGINE==True" {
    disable-tunnel: w1 -> [_ _]
    frame condition #0 (active) {
    }
    frame condition #1 {
      # "Call Quit LabVIEW if running as a built application."
      n194 = Quit LabVIEW() -> ()  [unwired: 1 in]
    }
  }
